vi "DAQ 1SDI v05.vi"() -> ()   [LabVIEW 2013]
uses:
  <instrlib>/niScope/Controls/niScope vertical coupling.ctl
  Strict Type Defs/type_meas_enum.ctl
  Strict Type Defs/Monitor switches.ctl
  Global VIs/shotnoise.vi
panel:
  in  "stop":bool
  in  "Monitors":T1(tab)=enum."Monitors On 2"
  out "Variance 1 normalised to SNL":dbl(graph)=-57.215073874003856
  out "Conditional variance":dbl(graph)=1.8987568233396978e-06
  out "Variance 2 normalised to SNL":dbl(graph)=-57.439490361932634
  out "covariance":dbl(graph)=-1.3543341759209789e-08
  out "covariance A|B":dbl(graph)=0.0015375102072466731
  out "Conditional variance A|B":dbl(graph)=1.007704030967265
  out "Key rate A|B":dbl(graph)=-0.4537670133032579
  out "Loop count":i32=20570
  in  "Settings":enum32{"Settings and Record", "Under the hood"}(tab)
  out "Video bandwidth (Hz)":dbl=1.4
  in  "Minimum sample rate (S/s)":dbl=14000000.0 format="%#_6p"
  in  "Reference position":dbl(slide)=50.0 scale=0.0..100.0
  in  "max time (s)":dbl=10.0 caption="Time to run (s)"
  in  "Channel parameters":T3(array[cluster])=[{"Channel name"="0", "Input impedance (Ohms)"=2, "Maximum input frequency (Hz)"=7000000.0, "vertical coupling"=1, "Probe attenuation"=1.0, "Vertical range (V)"=0.5, "Vertical offset"=0.0, "channel enabled"=TRUE}, {"Channel name"="1", "Input impedance (Ohms)"=2, "Maximum input frequency (Hz)"=7000000.0, "vertical coupling"=1, "Probe attenuation"=1.0, "Vertical range (V)"=0.5, "Vertical offset"=0.0, "channel enabled"=TRUE}] {"Input impedance (Ohms)" items=["1 mega ohm"=0, "50 ohms"=2]; "Maximum input frequency (Hz)" format="%#_6p"; "vertical coupling" items=["AC", "DC", "Ground"]}
  in  "IIR filter specifications":T4={"Topology"=enum."Butterworth", "Type"=enum."Bandpass", "Order"=6, "Lower Fc"=2900000.0, "Upper Fc"=3100000.0, "PB Ripple"=1.0, "SB Attenuation"=60.0} {"PB Ripple" format="%0.2f"; "SB Attenuation" format="%0.2f"; "Lower Fc" format="%0.2p"; "Upper Fc" format="%0.2p"}
  in  "File location":path=path "C:/ni-rt/LabVIEW Data/June26_2"
  in  "Type of measurement":T5
  in  "File root name":string="Real_05_"
  in  "Number of samples":i32=10000000 format="%.0p"
  in  "reset sn":bool
  in  "Shot noise start":bool
  out "error out":errorcluster caption="error out final"
  in  "Additional text":string="OPA 1 optical power set to 15mV on HD A.\nOPA 2 optical power set to 15mV on HD B.\nLocal oscillator is set to 5V on HD.\nParametric gain set to 15 for OPA 1.\nParametric gain set to 15 for OPA 2.\nVertical range set to 0.5V for both channels.\nSample rate set to 14MS/s.\nMax input freq set to7MHz.\nVisibility between OPA 1 & OPA 2 = 99.6\nVisibility between OPA 1 & L.O.B = 98.9\nVisibility between OPA 1 & L.O. A = 98.8\nBoth squeezers expected to produce -7dB/11dB.\nLoss on EPR B =10.9% (0.5dB) \n"
  in  "Record":bool
  in  "Number of Files":i32=2
  out "File count":i32=1
  out "Actual samples acquired ch 0":i32=10000000
  out "Actual samples acquired ch 1":i32=10000000
  out "SN loop count":i64=54
  out "SN":dbl[](array[numeric])=[0.005932295887867628, 0.005582591332430751]
  out "Parameters values file":string="PARAMETERS VALUES\r\rThursday, June 26, 2014\r6:14 PM\r\rMaster ch 0 <-> HD1 AC a-b\nMaster ch 1 <-> HD2 AC a-b\n\rSample rate : \rMaster : 14.285714E+6 Samples per second\rNumber of samples :\rMaster ch 0 : 10.000000E+6\rMaster ch 1 : 10.000000E+6\rFiles names : \rReal_05__shot_ParametersValues_10000000.txt\rReal_05__shot_mch01_20000000.txt\r\rOPA 1 optical power set to 15mV on HD A.\nOPA 2 optical power set to 15mV on HD B.\nLocal oscillator is set to 5V on HD.\nParametric gain set to 15 for OPA 1.\nParametric gain set to 15 for OPA 2.\nVertical range set to 0.5V for both channels.\nSample rate set to 14MS/s.\nMax input freq set to7MHz.\nVisibility between OPA 1 & OPA 2 = 99.6\nVisibility between OPA 1 & L.O.B = 98.9\nVisibility between OPA 1 & L.O. A = 98.8\nBoth squeezers expected to produce -7dB/11dB.\nLoss on EPR B =10.9% (0.5dB) \n"
  in  "DAQ Card":refnum<k15>="PXI1Slot7"
  in  "Monitor Switches":T6
  # "Variance won't be displayed until shot noise is taken"
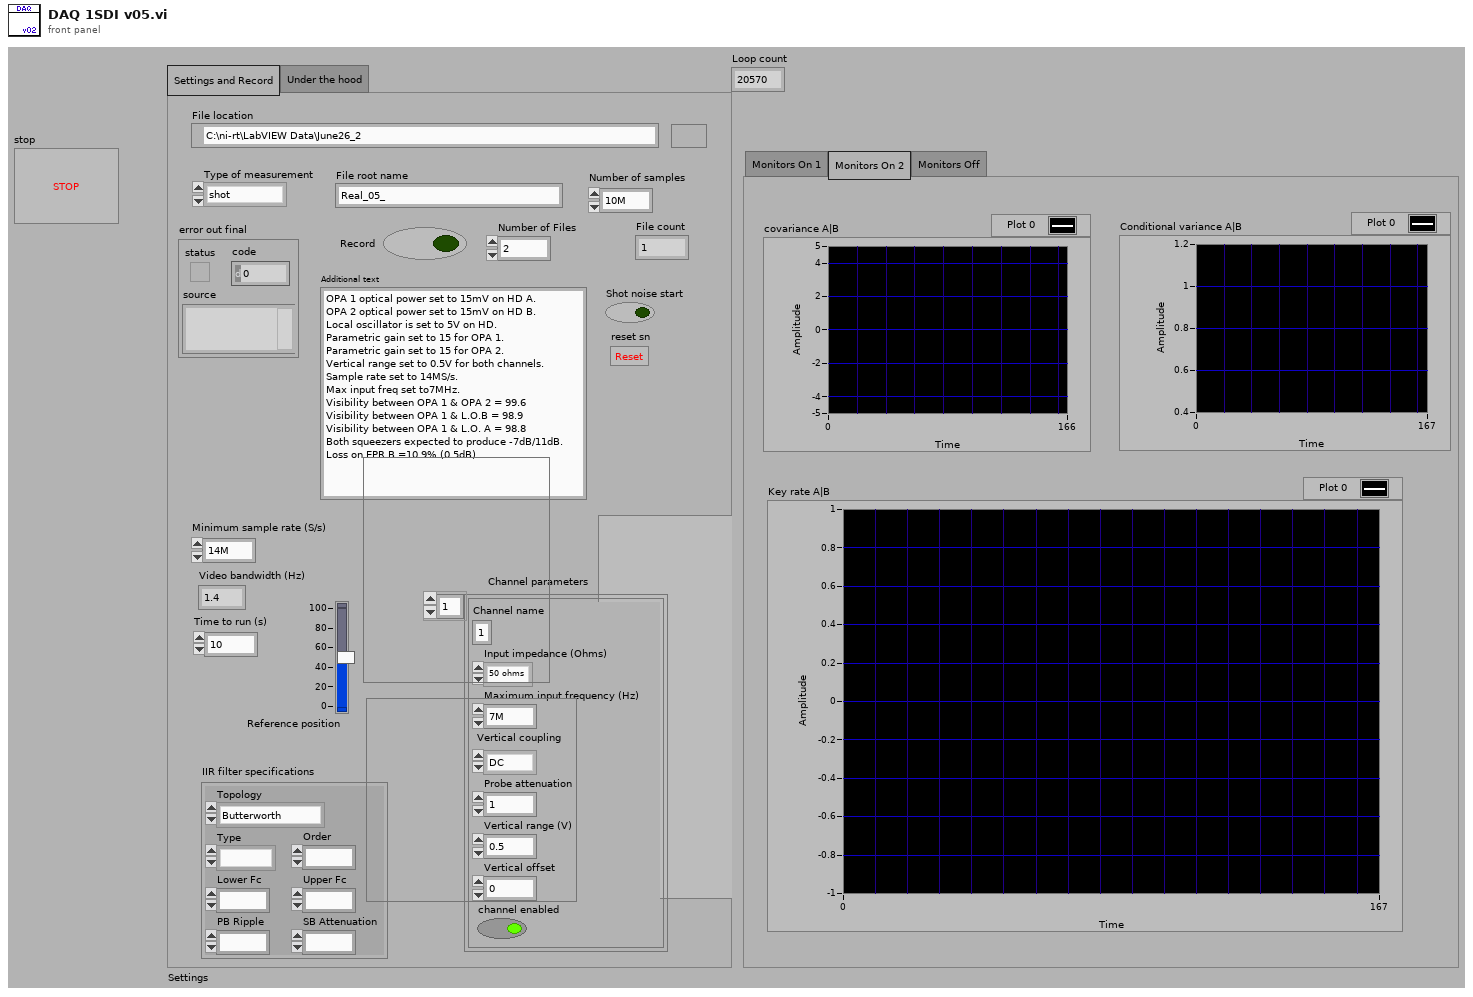
[diagram p1: front panel]
types:
  T1 = enum32{"Monitors On 1", "Monitors On 2", "Monitors Off"}
  T2 = typedef "niScope vertical coupling.ctl" = i32
  T3 = cluster{"Channel name":string, "Input impedance (Ohms)":u32, "Maximum input frequency (Hz)":dbl, "vertical coupling":T2, "Probe attenuation":dbl, "Vertical range (V)":dbl, "Vertical offset":dbl, "channel enabled":bool}[]
  T4 = cluster{"Topology":enum16{"Off", "Butterworth", "Chebyshev", "Inverse Chebyshev", "Elliptic", "Bessel"}, "Type":enum16{"Lowpass", "Highpass", "Bandpass", "Bandstop"}, "Order":i32, "Lower Fc":dbl, "Upper Fc":dbl, "PB Ripple":dbl, "SB Attenuation":dbl}
  T5 = typedef "type_meas_enum.ctl" = enum16{"shot", "x", "p", "electronic"}
  T6 = typedef "Monitor switches.ctl" = cluster{"Signal 1 On":bool, "Signal 2 On":bool, "Variance 1 On":bool, "Variance 2 On":bool, "Cov On":bool, "Cond. On":bool, "Monitors On":bool}
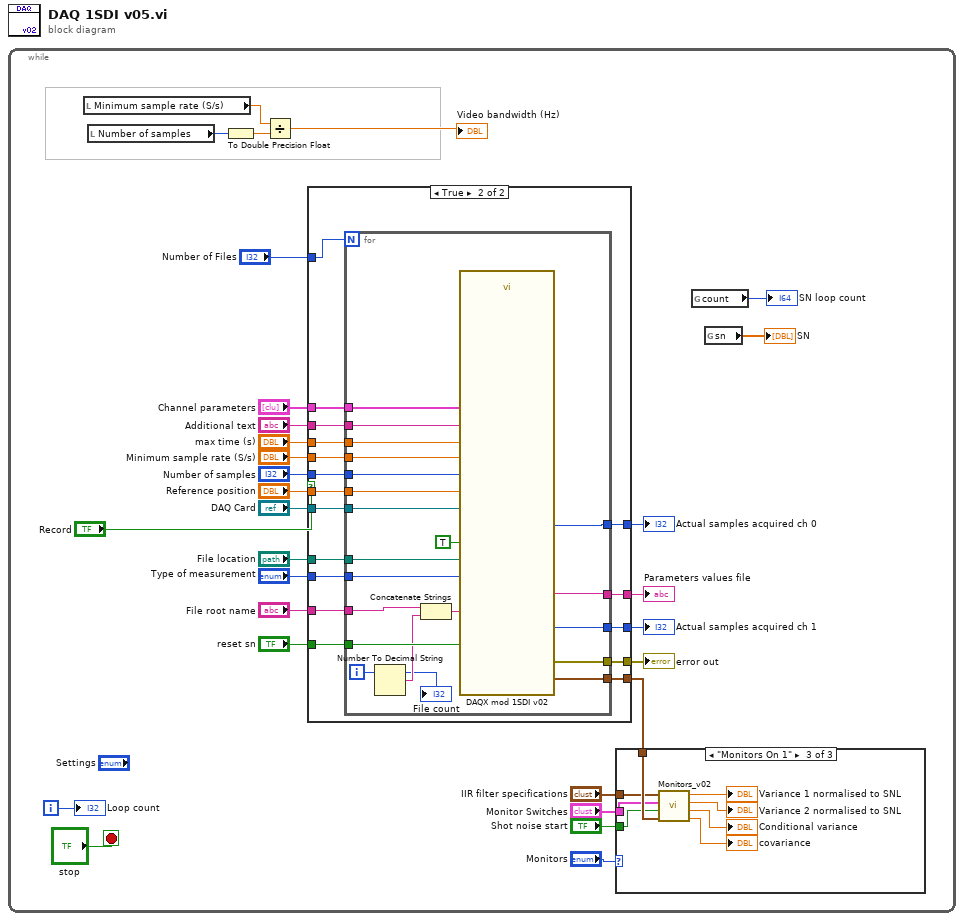
[diagram p0: block diagram]
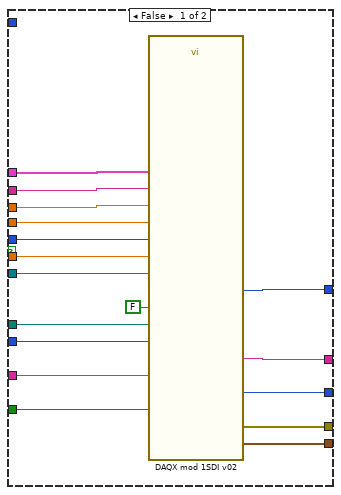
[diagram p2: hidden frame]
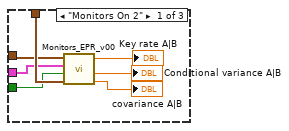
[diagram p3: hidden frame]
diagram:
  n1 = while {
    i -> [w14]
    stop <- "stop" stop-if-true
    n2 = local read "Minimum sample rate (S/s)"() -> (w28:dbl)
    n3 = local read "Number of samples"() -> (w30:i32)
    n4 = To Double Precision Float(number=w30) -> (double precision float=w27:dbl)
    n5 = Divide(x=w28, y=w27) -> (x/y=→"Video bandwidth (Hz)":dbl)
    n6 = case shown="True" "Record" {
      tunnel: "Channel parameters" -> [w46 w64]
      tunnel: "max time (s)" -> [w44 w63]
      tunnel: "Minimum sample rate (S/s)" -> [w43 w62]
      tunnel: "Reference position" -> [w41 w61]
      tunnel: "Number of samples" -> [w42 w60]
      tunnel: [w35 w59] -> w21
      tunnel: "DAQ Card" -> [w40 w58]
      tunnel: "File location" -> [w39 w57]
      tunnel: "Type of measurement" -> [w38 w56]
      tunnel: [w34 w55] -> w17
      tunnel: "File root name" -> [w36 w54]
      tunnel: [w33 w53] -> w15
      tunnel: [w32 w52] -> w11
      tunnel: [w31 w51] -> w10
      tunnel: "reset sn" -> [w37 w50]
      tunnel: "Additional text" -> [w45 w49]
      tunnel: "Number of Files" -> [_ w48]
      frame False {
        n7 = call "DAQX mod 1SDI v02.vi"("resource name"=w40, "Record Data"=FALSE, "numSamples"=w42, "max time (s)"=w44, "min sample rate"=w43, "File location"=w39, "reference position"=w41, "Additional text"=w45, "Type of measurement"=w38, "Name root"=w36, "channel parameters"=w46, "reset sn"=w37) -> ("wfm out"=w31:waveform(dbl)[], "Parameters values file"=w34:string, "actualSamples 0"=w35:i32, "actualSamples 1"=w33:i32, "error out"=w32:errorcluster)  [unwired: 11 in]
      }
      frame True {
        n8 = for {
          N: w48 -> [_]
          tunnel: w64 -> [w84]
          tunnel: w63 -> [w83]
          tunnel: w62 -> [w82]
          tunnel: w61 -> [w81]
          tunnel: w60 -> [w80]
          tunnel: [w79] -> w59
          tunnel: w58 -> [w78]
          tunnel: w57 -> [w77]
          tunnel: w56 -> [w76]
          tunnel: [w75] -> w55
          tunnel: w54 -> [w68]
          tunnel: [w74] -> w53
          tunnel: [w73] -> w52
          tunnel: [w72] -> w51
          tunnel: w50 -> [w71]
          tunnel: w49 -> [w70]
          i -> [w65]
          n9 = Number To Decimal String(number=w65) -> (decimal integer string=w66:string)  [unwired: 1 in]
          n10 = Concatenate Strings(w68, w66) -> (w67:string)
          n11 = call "DAQX mod 1SDI v02.vi"("resource name"=w78, "Record Data"=TRUE, "numSamples"=w80, "max time (s)"=w83, "min sample rate"=w82, "File location"=w77, "reference position"=w81, "Additional text"=w70, "Type of measurement"=w76, "Name root"=w67, "channel parameters"=w84, "reset sn"=w71) -> ("wfm out"=w72:waveform(dbl)[], "Parameters values file"=w75:string, "actualSamples 0"=w79:i32, "actualSamples 1"=w74:i32, "error out"=w73:errorcluster)  [unwired: 11 in]
          "File count" <- w65
        }
      }
    }
    "Actual samples acquired ch 0" <- w21
    "Parameters values file" <- w17
    "Actual samples acquired ch 1" <- w15
    "error out" <- w11
    n12 = case shown="\"Monitors On 1\"" "Monitors" {
      tunnel: w10 -> [w89 _ w99]
      tunnel: "IIR filter specifications" -> [w88 _ w94]
      tunnel: "Monitor Switches" -> [w87 _ w93]
      tunnel: "Shot noise start" -> [w86 _ w92]
      frame "Monitors On 2" {
        n13 = call "Monitors_EPR_v00.vi"("wfm"=w89, "Shot noise start"=w86, "Monitor Switches"=w87, "IIR filter specifications"=w88) -> ("covariance"=→"covariance A|B":dbl, "conditional variance A|B"=→"Conditional variance A|B":dbl, "Key Rate A|B"=→"Key rate A|B":dbl)  [unwired: 5 in]
      }
      frame "Monitors Off" {
      }
      frame "Monitors On 1" {
        n14 = call "Monitors_v02.vi"("wfm"=w99, "Shot noise start"=w92, "Monitor Switches"=w93, "IIR filter specifications"=w94) -> ("covariance"=→"covariance":dbl, "conditional variance"=→"Conditional variance":dbl, "Variance 2 normalised to SNL"=→"Variance 2 normalised to SNL":dbl, "Variance 1 normalised to SNL"=→"Variance 1 normalised to SNL":dbl)  [unwired: 4 in]
      }
    }
    n15 = global read "shotnoise.vi" "count"() -> (→"SN loop count":i64)
    n16 = global read "shotnoise.vi" "sn"() -> (→"SN":dbl[])
    "Loop count" <- w14
  }
